vi "To String.vi"(8 "error in (no error)":errorcluster, 11 "Types in":refnum<class "Abs_String 1D.lvclass">) -> (0 "error out":errorcluster, 2 "String":string, 3 "Types out":refnum<class "Abs_String 1D.lvclass">)   [LabVIEW 2021, in "Abs_String 1D.lvclass"]
uses:
  Abs_String 1D.lvclass
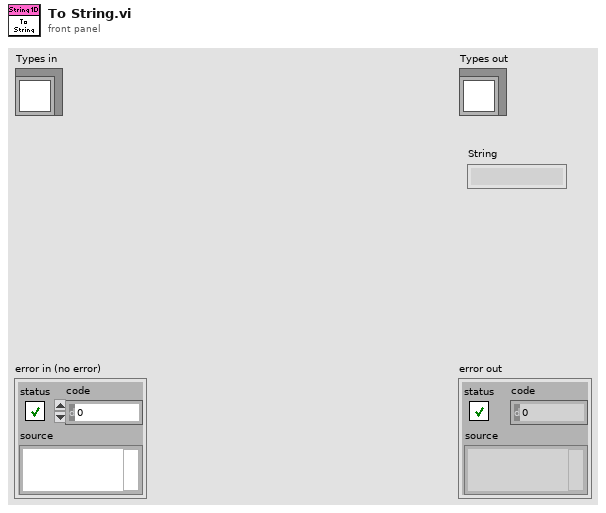
[diagram p1: front panel]
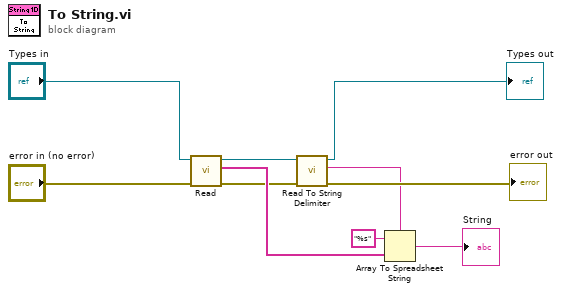
[diagram p0: block diagram]
diagram:
  n1 = call-dynamic "Read.vi"("error in (no error)"="error in (no error)", "Abs_String in"="Types in") -> ("error out"=w5:errorcluster, "Array"=w8:string[], "Abs_String out"=w4:refnum<class "Abs_String 1D.lvclass">)  [unwired: 7 in]
  n2 = call-dynamic "Read To String Delimiter.vi"("error in (no error)"=w5, "Abs_Array in"=w4) -> ("error out"=→"error out":errorcluster, "To String Delimiter"=w1:string, "Abs_Array out"=→"Types out":refnum<class "Abs_String 1D.lvclass">)  [unwired: 7 in]
  n3 = Array To Spreadsheet String(delimiter (Tab)=w1, array=w8, 3:"%s" ("format string")) -> (spreadsheet string=→"String":string)
